vi "SelectTeam.vi"() -> (2 "Selected Team":string(combo))   [LabVIEW 2017]
panel:
  in  "OK":bool
  in  "Select Team":string(combo)
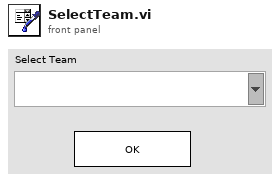
[diagram p1: front panel]
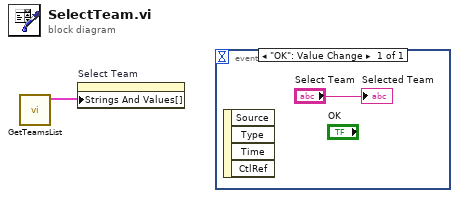
[diagram p0: block diagram]
diagram:
  n1 = call "GetTeamsList.vi"() -> ("Array"=w1:cluster{string, "value":string}[])  [unwired: 11 in]
  n2 = property on="Select Team" class="CmbBox"("Strings And Values[]"=w1) -> ()  [unwired: 2 in, 2 out]
  n3 = event shown="[0] \"OK\": Value Change" {
    selector: _ -> [_]
    dyn-events: _ -> [_]
    timeout: _ -> [_]
    event "OK": Value Change {
      n4 = event-data() -> ()  [unwired: 1 in, 4 out]
      "Selected Team" <- "Select Team"
    }
  }
